vi "Keithley 24XX Initialize.vi"(4 "error in (no error)":errorcluster, 7 "GPIB Address":refnum<visa-resource-name>="GPIB0::24::INSTR") -> (0 "error out":errorcluster, 2 "Instrument ID String":string, 3 "dup VISA Session":refnum<visa-resource-name>)   [LabVIEW 2020]
doc: "This VI Sets the parameters of the GPIB Interface for Re-Addressing, Assert REN and System controller. You must run this VI before using any of the instrument driver VIs for this instrument."
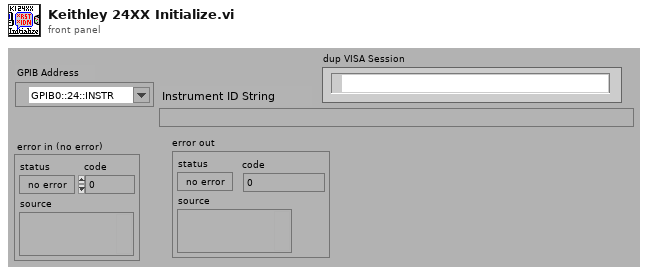
[diagram p1: front panel]
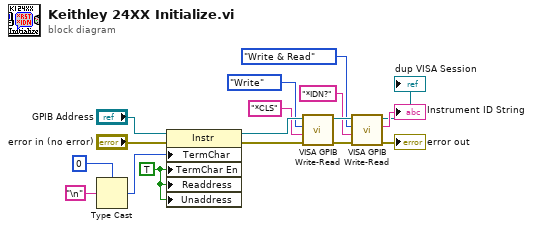
[diagram p0: block diagram]
diagram:
  w9 = TRUE
  n1 = Type Cast(type=u8 0 ("Message Based Settings:Termination Character"), x="\n") -> (*(type *) &x=w13:u8)
  n2 = property class="Instr"(reference="GPIB Address", error in="error in (no error)", "TermChar"=w13, "TermChar En"=w9, "Readdress"=w9, "Unaddress"=w9) -> (reference out=w16:refnum<visa-resource-name>, error out=w11:errorcluster)
  n3 = call "VISA GPIB Write-Read.vi"("error in (no error)"=w11, "Command"="*CLS", "Action"=enum16{"Write", "Read", "Write & Read"}."Write", "VISA resource name"=w16) -> ("error out"=w7:errorcluster, "dup VISA Session"=w8:refnum<visa-resource-name>)  [unwired: 4 in, 2 out]
  n4 = call "VISA GPIB Write-Read.vi"("error in (no error)"=w7, "Command"="*IDN?", "Action"=enum16{"Write", "Read", "Write & Read"}."Write & Read", "VISA resource name"=w8) -> ("error out"=→"error out":errorcluster, "String Returned"=→"Instrument ID String":string, "dup VISA Session"=→"dup VISA Session":refnum<visa-resource-name>)  [unwired: 4 in, 1 out]
